vi "Unflatten From String to Variant with Attributes.vi"(8 "error in (no error)":errorcluster, 10 "String":string, 11 "Deserializer in":refnum<class "JSON Deserializer.lvclass">) -> (0 "error out":errorcluster, 2 "Variant with Attributes":variant, 3 "Deserializer out":refnum<class "JSON Deserializer.lvclass">)   [LabVIEW 2015, in "JKI JSON Serialization.lvlib" / "JSON Deserializer.lvclass"]
doc: "Converts a JSON formatted <b>String</b> to <b>Variant</b>. If <b>Type and Defaults</b> is provided, converts JSON string to the specified type if the type is compatible with the value of the JSON string. For any cluster element in Type and Defaults, the value of the element in Type and Default is used if element with the same name is not present in the JSON string."
uses:
  JSON Deserializer.lvclass
  JSON Parser/JSON Parser.lvclass
  <vilib>/Utility/Data Type/NI_Data Type.lvlib
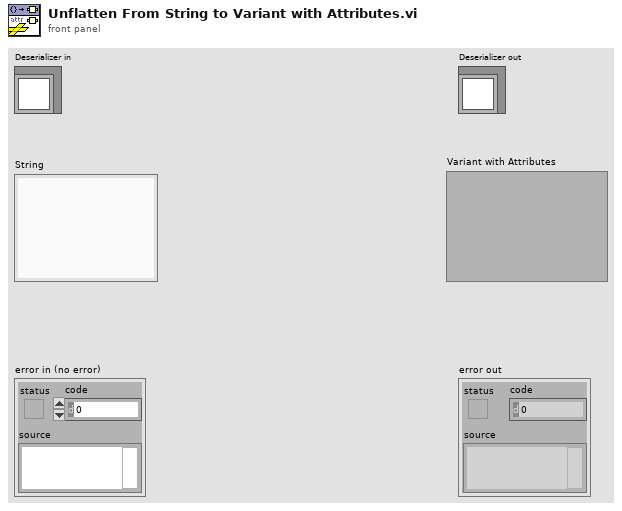
[diagram p1: front panel]
types:
  T1 = typedef "NI_Data Type.lvlib/Data Type.ctl" = enum8{"Invalid Type", "Void", "I8", "I16", "I32", "I64", "U8", "U16", "U32", "U64", "Single Float", "Double Float", "Extended Float", "Single Complex", "Double Complex", "Extended Complex", "Enum U8", "Enum U16", "Enum U32", "Enum U64", "Single Float With Unit", "Double Float With Unit", "Extended Float With Unit", "Single Complex with Unit", "Double Complex with Unit", "Extended Complex with Unit", "Boolean", "String", "Path", "Picture", "Tag", "Array", "Cluster", "Variant", "LV Variant", "Waveform", "Timestamp", "Digital Waveform", "Digital Data", "ExpressData", "Refnum", "External Data", "VI", "Poly VI", "LabVIEW Class Instance", "Fixed Point"}
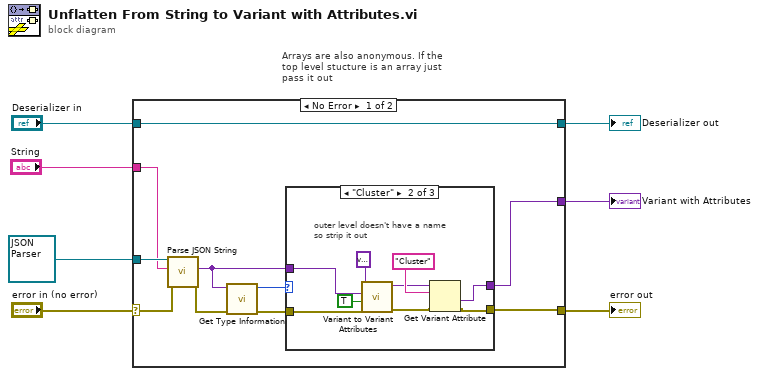
[diagram p0: block diagram]
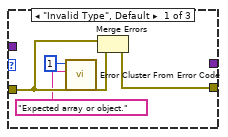
[diagram p2: hidden frame]
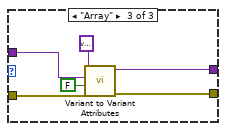
[diagram p3: hidden frame]
diagram:
  # "Arrays are also anonymous. If the\ntop level stucture is an array just\npass it out"
  n1 = case shown="No Error" "error in (no error)" {
    selector: "error in (no error)" -> [w16 w38]
    tunnel: "Deserializer in" -> [w14 w39]
    tunnel: refnum<class "JSON Parser.lvclass"> refnum ("Alpaca CLI Command Parser in") -> [w17 _]
    tunnel: "String" -> [w15 _]
    tunnel: [w13 w38] -> w3
    tunnel: [w14 w39] -> w2
    tunnel: [w12 _] -> w1
    frame No Error {
      n2 = call-dynamic "Parse JSON String.vi"("error in (no error)"=w16, "Parse Argument String"=w15, "Alpaca CLI Command Parser in"=w17) -> ("error out"=w11:errorcluster, "Value"=w8:variant)  [unwired: 6 in, 1 out]
      n3 = call <vilib>:"Get Type Information.vi"("error in (no error)"=w11, "Variant"=w8) -> ("error out"=w10:errorcluster, "Type"=w9:T1)  [unwired: 5 in, 3 out]
      n4 = case shown="\"Cluster\"" w9 {
        tunnel: w8 -> [_ w30 w36]
        tunnel: [w20 w25 w35] -> w13
        tunnel: [_ w23 w33] -> w12
        tunnel: w10 -> [w22 w28 w32]
        frame "Invalid Type", Default {
          n5 = call <vilib>:"Error Cluster From Error Code.vi"("error in (no error)"=w22, "error message (\"\")"="Expected array or object.", "error code (0)"=1) -> ("error out"=w21:errorcluster)  [unwired: 6 in]
          n6 = Merge Errors(w22, w21) -> (w20:errorcluster)
        }
        frame "Cluster" {
          # "outer level doesn't have a name\nso strip it out"
          n7 = call "Variant to Variant Attributes.vi"("error in"=w28, "Parent is object"=TRUE, "Variant"=w30, "Variant with Attributes"=variant) -> ("error out"=w26:errorcluster, "Variant with Attributes"=w24:variant)  [unwired: 6 in]
          n8 = Get Variant Attribute(Variant=w24, name="Cluster", error in=w26) -> (value=w23:variant, error out=w25:errorcluster)  [unwired: 1 in, 2 out]
        }
        frame "Array" {
          n9 = call "Variant to Variant Attributes.vi"("error in"=w32, "Parent is object"=FALSE, "Variant"=w36, "Variant with Attributes"=variant) -> ("error out"=w35:errorcluster, "Variant with Attributes"=w33:variant)  [unwired: 6 in]
        }
      }
    }
    frame Error {
    }
  }
  "error out" <- w3
  "Deserializer out" <- w2
  "Variant with Attributes" <- w1
